vi "Unit Test slice flattened object data on error False.vi"() -> ()   [LabVIEW 2019, in "Sports Unit Tests.lvclass"]
uses:
  Sports Unit Tests.lvclass
  Classes/Sports Player/Sports Player.lvclass
  <userlib>/Blue Origin/BlueSerialization/BlueSerializer/DeserializeOptions.ctl
  <userlib>/Blue Origin/BlueSerialization/BlueSerializer/DeserializeSlicingOptions.ctl
  <userlib>/Blue Origin/BlueSerialization/BlueSerializer/DeserializeMutationOptions.ctl
  <userlib>/Blue Origin/BlueSerialization/BlueSerializer/DeserializePreservationOptions.ctl
  <userlib>/Blue Origin/BlueSerialization/BlueSerializer/PreserveNonWiredDataOption.ctl
  <vilib>/Utility/error.llb/Clear Errors.vi
  <vilib>/addons/_JKI Toolkits/Caraya/classes/Test/Define Test.vi
  <vilib>/addons/_JKI Toolkits/Caraya/classes/Assert/Assert Equal Value_Variant.vi
  <vilib>/addons/_JKI Toolkits/Caraya/classes/Assert/Assert Error.vi
  <vilib>/addons/_JKI Toolkits/Caraya/classes/Assert/Assert.lvclass
  Classes/Tiger Woods/Tiger Woods.lvclass
  <userlib>/Blue Origin/BlueSerialization/BlueSerializer/BlueSerializer.lvclass
panel:
  out "Table":string[][](table)=[["{\r  \"Class\":[\"Tyler Durden.lvclass\",\"Golf Player.lvclass\",\"Sports Player.lvclass\",\"Human.lvclass\",\"BlueSerialization.lvlib:BlueSerializable.lvclass\"],\r  \"Version\":[\"2.0.0.3\",\"2.0.0.3\",\"2.0.0.3\",\"2.0.0.3\",\"2.0.0.0\"],\r  \"BlueSerialization.lvlib:BlueSerializable.lvclass\":{\"LibVersion\":1},\r  \"Human.lvclass\":{\r    \"alive?\":true,\r    \"Age (years)\":31,\r    \"Name\":\"Tiger\",\r    \"Height (ft)\":6\r  },\r  \"Sports Player.lvclass\":{\r    \"Professional?\":true,\r    \"Earnings (dollars)\":1000000,\r    \"Sponsor\":\"Monster Energy\"\r  },\r  \"Golf Player.lvclass\":{\r    \"League\":\"PGA\",\r    \"# holes in one\":30,\r    \"longest drive (ft)\":3000\r  },\r  \"Tyler Durden.lvclass\":{\r    \"Current tour\":\"Worlds\",\r    \"# tantrums thrown\":99\r  }\r}", "{\r  \"Class\":[\"BlueSerialization.lvlib:BlueSerializable.lvclass\"],\r  \"Version\":[\"2.0.0.0\"],\r  \"BlueSerialization.lvlib:BlueSerializable.lvclass\":{\"LibVersion\":0}\r}", "Status: TRUE\ncode: 1373\nFailed in instantiate child class from class name specified in the serialized text.\nTurn on \"Allow class slicing upwards\" to allow for Serializer to recurse upwards until finding the first available parent in memory for which to instantiate.\nChild class: \"Tyler Durden.lvclass\"Get LV Class Default Value By Name.vi<APPEND>\n\n<b>Complete call chain:</b>\r\n     Get LV Class Default Value By Name.vi\r\n     BlueSerialization.lvlib:BlueSerializer.lvclass:GetLVObject.vi:4550001\r\n     BlueJSONTextSerializer.lvlib:BlueJSONTextSerializer.lvclass:LVObject Callback.vi:70004\r\n     BlueJSONtext.lvlib:JSON text to Variant.vi:4410001\r\n     BlueJSONTextSerializer.lvlib:BlueJSONTextSerializer.lvclass:TextToVariant.vi:3020001\r\n     BlueSerialization.lvlib:BlueSerializer.lvclass:Deserialize.vi:7360001\r\n     Sports Unit Tests.lvclass:Unit Test Allow Class Slicing On Deserialize ALL False.vi\r\n\r\n<b>LabVIEW attempted to find the class with this name:</b>\r\nTyler Durden.lvclass", "BlueJSONTextSerializer.lvlib:BlueJSONTextSerializer.lvclass"], ["Class = [\"Tyler Durden.lvclass\", \"Golf Player.lvclass\", \"Sports Player.lvclass\", \"Human.lvclass\", \"BlueSerialization.lvlib:BlueSerializable.lvclass\"]\r\nVersion = [\"2.0.0.3\", \"2.0.0.3\", \"2.0.0.3\", \"2.0.0.3\", \"2.0.0.0\"]\r\n\n[\"BlueSerialization.lvlib:BlueSerializable.lvclass\"]\nLibVersion = 1\r\n\n[\"Human.lvclass\"]\n\"alive?\" = true\r\n\"Age (years)\" = 31\r\nName = \"Tiger\"\r\n\"Height (ft)\" = 6.0\r\n\n[\"Sports Player.lvclass\"]\n\"Professional?\" = true\r\n\"Earnings (dollars)\" = 1000000.0\r\nSponsor = \"Monster Energy\"\r\n\n[\"Golf Player.lvclass\"]\nLeague = \"PGA\"\r\n\"# holes in one\" = 30\r\n\"longest drive (ft)\" = 3000.0\r\n\n[\"Tyler Durden.lvclass\"]\n\"Current tour\" = \"Worlds\"\r\n\"# tantrums thrown\" = 99\r\n", "Class = [\"BlueSerialization.lvlib:BlueSerializable.lvclass\"]\r\nVersion = [\"2.0.0.0\"]\r\n\n[\"BlueSerialization.lvlib:BlueSerializable.lvclass\"]\nLibVersion = 0\r\n", "Status: TRUE\ncode: 1373\nFailed in instantiate child class from class name specified in the serialized text.\nTurn on \"Allow class slicing upwards\" to allow for Serializer to recurse upwards until finding the first available parent in memory for which to instantiate.\nChild class: \"Tyler Durden.lvclass\"Get LV Class Default Value By Name.vi<APPEND>\n\n<b>Complete call chain:</b>\r\n     Get LV Class Default Value By Name.vi\r\n     BlueSerialization.lvlib:BlueSerializer.lvclass:GetLVObject.vi:4550001\r\n     BlueTOMLSerializer.lvlib:TOML to LabVIEW.vi:3370001\r\n     BlueTOMLSerializer.lvlib:BlueTOMLSerializer.lvclass:TextToVariant.vi:3020001\r\n     BlueSerialization.lvlib:BlueSerializer.lvclass:Deserialize.vi:7360001\r\n     Sports Unit Tests.lvclass:Unit Test Allow Class Slicing On Deserialize ALL False.vi\r\n\r\n<b>LabVIEW attempted to find the class with this name:</b>\r\nTyler Durden.lvclass", "BlueTOMLSerializer.lvlib:BlueTOMLSerializer.lvclass"]]
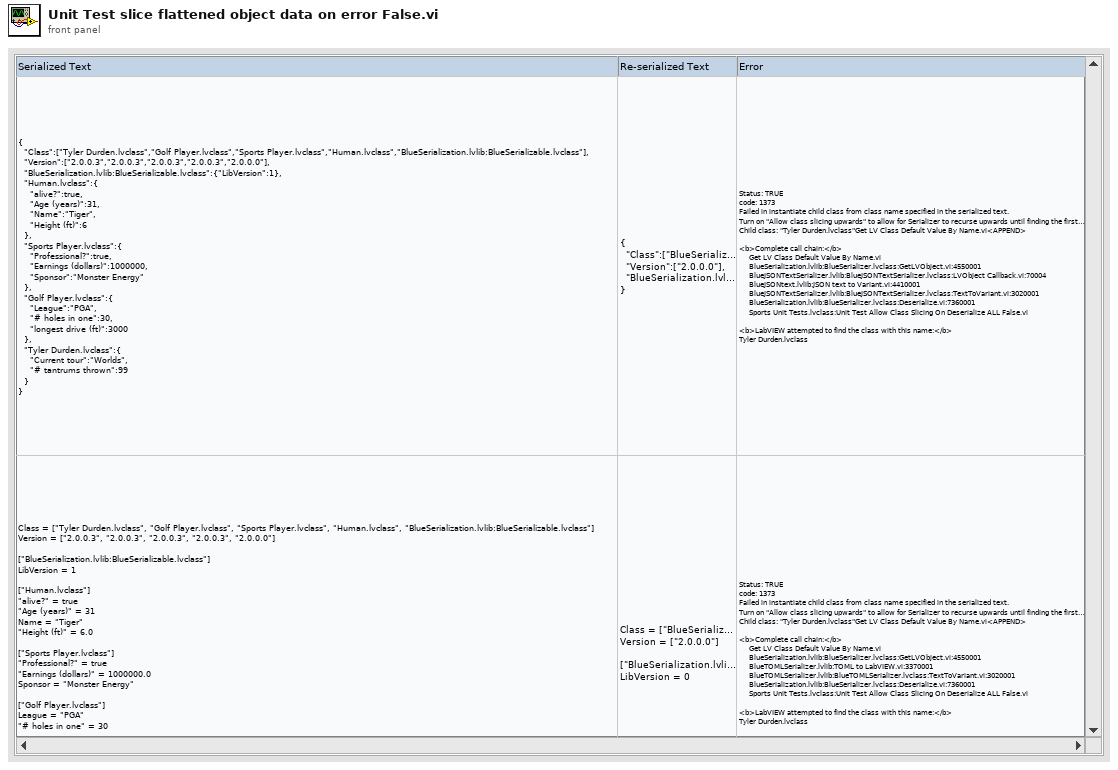
[diagram p1: front panel]
types:
  T1 = typedef "BlueSerialization.lvlib/BlueSerializer.lvclass/DeserializeOptions.ctl" = cluster{"deserialize non-BlueSerializable objects from hex?":bool, "expand objects on type conflict?":bool, "Slicing":T2, "Mutation Options":T3, "Preservation Options":T4}
  T2 = typedef "BlueSerialization.lvlib/BlueSerializer.lvclass/DeserializeSlicingOptions.ctl" = cluster{"slice flattened object data on error?":bool, "sliceable class names":string[]}
  T3 = typedef "BlueSerialization.lvlib/BlueSerializer.lvclass/DeserializeMutationOptions.ctl" = cluster{"error on inserted parent levels?":bool, "\terror on obsolete parent levels?":bool}
  T4 = typedef "BlueSerialization.lvlib/BlueSerializer.lvclass/DeserializePreservationOptions.ctl" = cluster{"Preserve wired serialized data?":bool, "Preserve wired non-serialized data":T5}
  T5 = typedef "BlueSerialization.lvlib/BlueSerializer.lvclass/PreserveNonWiredDataOption.ctl" = enum16{"Don't preserve", "Preserve (error on less-specific wired types)", "Preserve (except on less-specific wired types)"}
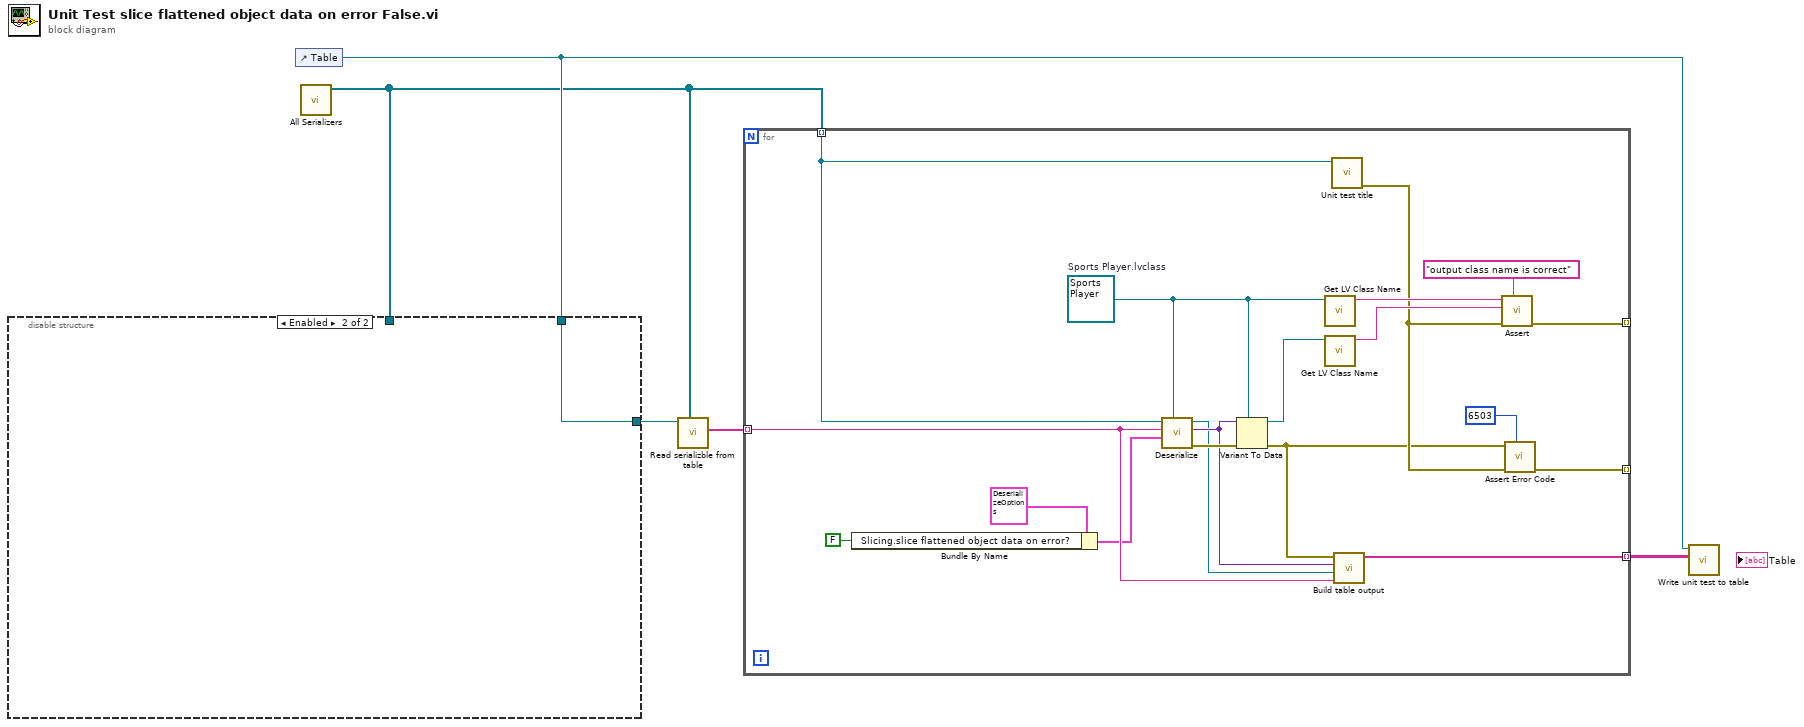
[diagram p0: block diagram]
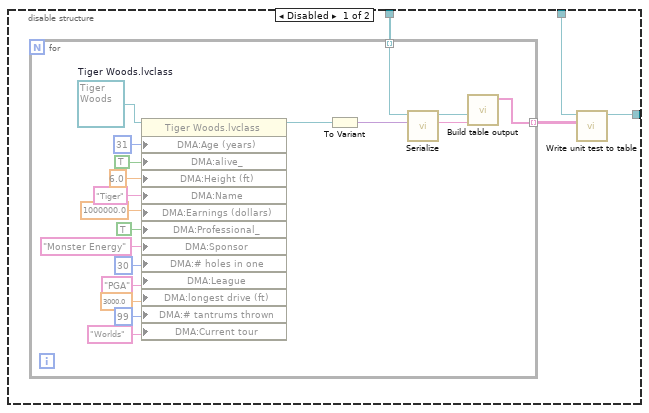
[diagram p2: hidden frame]
diagram:
  n1 = control-ref of="Table"() -> (w5:refnum<vi>)
  n2 = call "All Serializers.vi"() -> ("All serializers"=w2:refnum<class "BlueSerializer.lvclass">[])  [unwired: 11 in]
  n3 = disable-structure "Diagram Disable Structure" shown="Enabled" {
    disable-tunnel: w5 -> [w8 w29]
    disable-tunnel: [w7 w29] -> w4
    disable-tunnel: w2 -> [w6 _]
    frame Disabled {
      n4 = for {
        tunnel: w6 -> [w13] mode=indexing
        tunnel: [w10] -> w9 mode=indexing
        w23 = refnum<class "Tiger Woods.lvclass"> refnum  # Tiger Woods.lvclass
        n5 = property on="Property Node" class="Tiger Woods.lvclass"(reference=w23, "DMA:Age (years)"=u16 31 ("Age (years)"), "DMA:alive_"=TRUE ("alive_"), "DMA:Height (ft)"=6.0 ("Height (ft)"), "DMA:Name"="Tiger" ("Name"), "DMA:Earnings (dollars)"=1000000.0 ("Earnings (dollars)"), "DMA:Professional_"=TRUE ("Professional_"), "DMA:Sponsor"="Monster Energy" ("Sponsor"), "DMA:# holes in one"=30 ("# holes in one"), "DMA:League"="PGA" ("League"), "DMA:longest drive (ft)"=3000.0 ("longest drive (ft)"), "DMA:# tantrums thrown"=99 ("# tantrums thrown"), "DMA:Current tour"="Worlds" ("Current tour")) -> (reference out=w22:refnum<class "Tiger Woods.lvclass">)  [unwired: 1 in, 1 out]
        n6 = To Variant(anything=w22) -> (Variant=w14:variant)
        n7 = call <userlib>:"Serialize.vi"("Anything"=w14, "BlueSerializer in"=w13) -> ("Serialized Text"=w11:string, "BlueSerializer out"=w12:refnum<class "BlueSerializer.lvclass">)  [unwired: 7 in, 1 out]
        n8 = call "Build table output.vi"("serialized text"=w11, "BlueSerializer in"=w12) -> ("table output"=w10:string[])  [unwired: 9 in]
      }
      n9 = call "Write unit test to table.vi"("Table"=w9, "Table ref in"=w8) -> ("Table ref out"=w7:refnum<vi>)  [unwired: 9 in]
    }
    frame Enabled {
    }
  }
  n10 = call "Read serializble from table.vi"("serializers"=w2, "Table ref in"=w4) -> ("serializable texts"=w3:string[])  [unwired: 7 in, 2 out]
  n11 = for {
    tunnel: w2 -> [w31] mode=indexing
    tunnel: [w41] -> _ mode=indexing
    tunnel: [w43] -> _ mode=indexing
    tunnel: w3 -> [w35] mode=indexing
    tunnel: [w34] -> w1 mode=indexing
    w39 = refnum<class "Sports Player.lvclass"> refnum  # Sports Player.lvclass
    n12 = Bundle By Name(cluster=T1 {"deserialize non-BlueSerializable objects from hex?"=FALSE, "expand objects on type conflict?"=FALSE, "Slicing"={"slice flattened object data on error?"=FALSE, "sliceable class names"=[]}, "Mutation Options"={"error on inserted parent levels?"=FALSE, "\terror on obsolete parent levels?"=FALSE}, "Preservation Options"={"Preserve wired serialized data?"=FALSE, "Preserve wired non-serialized data"=enum."Don't preserve"}} ("Deserialize Options"), "Slicing.slice flattened object data on error?"=FALSE ("Allow class expansion?")) -> (w30:T1)
    n13 = call <userlib>:"Deserialize.vi"("Anything"=w39, "Deserialize Options"=w30, "Serialized Text"=w35, "BlueSerializer in"=w31) -> ("error out"=w48:errorcluster, "Variant"=w37:variant, "BlueSerializer out"=w36:refnum<class "BlueSerializer.lvclass">)  [unwired: 5 in]
    n14 = Variant To Data(error in=w48, type=w39, Variant=w37) -> (data=w47:refnum<class "Sports Player.lvclass">, error out=w38:errorcluster)
    n15 = call <vilib>:"Get LV Class Name.vi"("object"=w39) -> ("class name"=w46:string)  [unwired: 9 in, 1 out]
    n16 = call <vilib>:"Get LV Class Name.vi"("object"=w47) -> ("class name"=w45:string)  [unwired: 9 in, 1 out]
    n17 = call "Unit test title.vi"("serializer"=w31) -> ("error out"=w42:errorcluster)  [unwired: 9 in, 1 out]
    n18 = call "Build table output.vi"("serialized text"=w35, "BlueSerializer in"=w36, "deserialized variant"=w37, "variant to data error"=w38) -> ("table output"=w34:string[])  [unwired: 7 in]
    n19 = call-poly <vilib>:"Assert.vi"("Label"="output class name is correct", "error in (no error)"=w42, "Y"=w45, "X"=w46) -> ("error out"=w43:errorcluster)  [unwired: 7 in]
    n20 = call "Assert Error Code.vi"("Assert specific error code"=6503, "error in (no error)"=w42, "Error?"=w38) -> ("error out"=w41:errorcluster)  [unwired: 8 in]
  }
  n21 = call "Write unit test to table.vi"("Table"=w1, "Table ref in"=w5) -> ()  [unwired: 9 in, 1 out]
